vi "Main_24b.vi"() -> ()   [LabVIEW 2020]
uses:
  RB ENUM_Position ID.ctl
  Cluster _Point Location.ctl
  0c90424e-a446-4045-a5ae-fd3bd7481f50.vi
  <vilib>/Comparison/Equal/Equal Functor/Equal Functor.lvclass
panel:
  in  "milliseconds to wait":u32
  in  "Description":string="--- Part Two ---\nAs the expedition reaches the far side of the valley, one of the Elves looks especially dismayed:\n\nHe forgot his snacks at the entrance to the valley!\n\nSince you're so good at dodging blizzards, the Elves humbly request that you go back for his snacks. From the same initial conditions, how quickly can you make it from the start to the goal, then back to the start, then back to the goal?\n\nIn the above example, the first trip to the goal takes 18 minutes, the trip back to the start takes 23 minutes, and the trip back to the goal again takes 13 minutes, for a total time of 54 minutes."
  out "Array":T1[][](array[typedef])
  in  "Example 2":string="#.######\n#>>.<^<#\n#.<..<<#\n#>v.><>#\n#<^v^^>#\n######.#"
  out "Answer":i32
  in  "Puzzle":string="#.######################################################################################################################################################\n#>v<<.^vvv^vv.^^>>v<>><v^<<.>^>v>v<v^vvvvvv^><^<vv<^^^v<vv>vvv.^v>.<>>v^v><<>^<<^vv<<>><<v<v<^v<..^>>vv^><<<v<^^><<<>>>vvv^.^.v>.^v^^.vv>^vv^>^^^><v<<<#\n#.<<v^><<.<>>>>^.<^<^^<>>^.^^.^v<vvv>>vv<^>.>>^^<<<^^>><^><<<v^>v.^^<.<<^v^>^^>.^.v^>.><<vv^>><>^....^<vv^><<^>v<v<^vvv<v<<><^vv<^>v^^^^^^^.^vv<^^<vvv<#\n#<>.v^.v<^><><v^^>>^><.v>^v^vv><><>>^>^v<^>>v^>^vvv^v..>vv>.^vv^<^.<.<v>>^<><v>^>^v..^>^><>vvv<v>^.>>^^<v^v>^<^vv.>.^v><v>v^>.^v<v>.<<vvv><^v^<^<^<vv<>#\n#>v..v^<^^v<><^^>vv>v^^^<^.^<<><^^^v>^<^v<<^>^<<.^><<^>>v^.v.><>>^<<><^^>>v>.^<^<vv><<>..>>v^^^>v>^<vv>.^>^<.^^v<>v>^.^>^^>.^v^>>^v>>>^<<^.^>><>v^>v>v.#\n#>^^^^^v^>>>^^v^v^v>v^v<v^.><<.^..v<^<^<^><<><<<>>v<<>><<^v^^>v>v<>.<vv>^<<<><.v<v<>>v^v<>>^v><.v>><<v><v<vv<<^^<><.^>v>^<^<^>^^.<.v>v^>>>><<<^v.vv<.<>#\n#>vv<vv^v<.<<v><<<^v>v<><vv<<vv<<.^.v>>v>.>v<^<<>v>>vv>..>v<^.v<.^<.>.<<<>>>^v>.^>>>>><<<^>..>>>^<^<>^>><>^><><v>v<<<v^.vvvv<v>>vv^>>>^.v^<>^><.<v>>v>>#\n#>>v.>><v^>v^v.<^.<vvv<<<v<>.^^v<<^^>>^^v^^.^.<>^vv^>>v<>^>v^.vv^v>.v^<>>v<<v<^>^vv^^v^><>v>.^<v<v<.^>>vvv>v^<^vv^<v^<<>^<v<>v<<v<<>v^v><>^vv^<<<^v>^>>#\n#<^<^>><<.<<.><<v>vv>v^v<<>..v<^>v^<.vv><v^<<<.v>v>>><<^.<v^vvv^<^v<<^^^^<v<<.<<^><v.<>>^><v>..<><vvv<.<>><.v>.v><<>vv<>.<<v.>><>>v<v^>^>>..>.<<^>^>^.>#\n#<v.>v>v<>>v^v>^v<^vv>^^>^vv>v<^^vv><^.<v<^<v>^>^v<v.<^<>^>>>vvvv<v>>^^<v.^v<^^<.<<<><v^<>^^<vvv><<>...^<><>^>vvv^^v..v..v^><^<>^>vv><v<^^vv^vvv>v^<v><#\n#<^^^^.>v>><<>v<vv<^<<^>v..vv^vvv>>>v<<^vv^^><^>^>^v.<<^v^^><vv>.>v..v.^v><^<^>>^>vv<<v.v>.<.>^.>>>^>>^^v^>^<.<><v>v^.^..<>.>^<^^<v.^v>^^^<<^v>>.>vv<v>#\n#>^^v>v.<v<<v..>><>..^v><>.^<v.>vv<>v^^>v.^v<<<vv>>v.^>><<^<v><v^.>>>^v>^>>v<<...<^^^vv.v^><<<>^^v<v^>v<v>.vv^vv.>>v<>><>v><vv>^>>v^..vv>v>^^>vvv>.>^v<#\n#<v>^^.<.^vv^<>^vv<<<<<vv^<^^<>v>^vv<>v<<>vv^<<v><<.^^..>.^>vv<^<>>^.<<<<<>.v>v><>.>v>v^<>^>vvv>.<^v^.>^<<v<^vvv^>v><<v^>.^><^><>v.^^<><vv<>.v..^<<v^>>#\n#<>^.>.><><v^<v>v>^<<>^v..<.<><>>^.vv>v.vv.>><>v^>.^><.<v.>v..^^v.^v^>^<^^<>>>v<^>>v<^<v^^^v<^v.vv<v^.><^^v^>^^^<.>.<v<.<v>^.><^^<v^<<^^v<.>>v>.vvv>v>>#\n#<v><v.^^<>v>.>^^^^>v<<v..v>><>v^.>^^<^>v<>v^v<v^<><^<>v>v^.<.^v^<^<>v^^<<^v><^.>^.v><><>>^v^v><.>v><<>v>v^.vvv><>^>>v^<<^v>^vv><><.^^>>vv^^v><^..>^v<>#\n#>v><^<vv^v>v><>v^<<><<^>v^v<^<^<v>><v^vv<<.vv<^v.><<<v.v.^<v<v.^^>><>^vv>v<v^>v^.<<><^<<.<vv<^.^>^^vv<^vv^..<^>^^<^^vvvv<><^^^<v<vv<v^>^v<^v><^^<..<v>#\n#>v^<<><<<^v.vvv>v<<v>>.^>^<^><..>>>^v.v.<<v<>>^^..><<v>vv^^<v<<^<>^v<^<<^.v>^<^>vv.>>>^>^^.<^<v<<^^v^^<><.>^.<><vv^<^>^>>^^vv^<^^^<^>^.v^<.<^^<.>v>v>>#\n#>^<v>v^<^>>..v<.><<<^><^v>vv<>^^v<v^vv><<<><^v<^.v<^>v<v<^<v>v>^v^^>>^<<^.<<v<vvv><^>v>^<>v>v^^>.<vv<<>>^^<>vv>^v^.><^^^vv>v<<<<v^v<vv><.<v<^v>>^v>v<>#\n#<vv^>^^<v>^v>>.^.<<^<^^.v>>vv>^<><><>>^>>>vv<.v<^<<<vvv.>v<>>^>>v<>>..>^v^>^>^v<<>v^v^.^>^v^^v>.><v<<.v<v>vv>>.<<v.v.^<>><>vv>^^>><^^.<>>>vv<<>^>><<<.#\n#<^<^^.>>>^<>^v<^v<<>v^<>^vv<^^v<v<<^^.><<vv>v^<^^<>^^^v<v>^.^^<<^v<v^.^>>>><v>><>>>><v<^^<v>v^v>^>v>v^^^<>v><v><.>><>^vvvvv>vv<<v^^<v^v>v.^v<vv<^.^^v<#\n#..>^>>^^^^v<>>^><^^v>^^>v.><>><vv<><^.<><^v.^vv<><v>v^<<v>v<vv<><>v^.^<<<vv>>^^<<>^.v<^.v^^<>>>^v<.>^..^^^<<<>..v<><v<>v<>>..<v><>^^>>.<>v<<>v>.<v^vv.#\n######################################################################################################################################################.#"
  in  "Example":string="#.#####\n#.....#\n#>....#\n#.....#\n#...v.#\n#.....#\n#####.#"
  # "976"
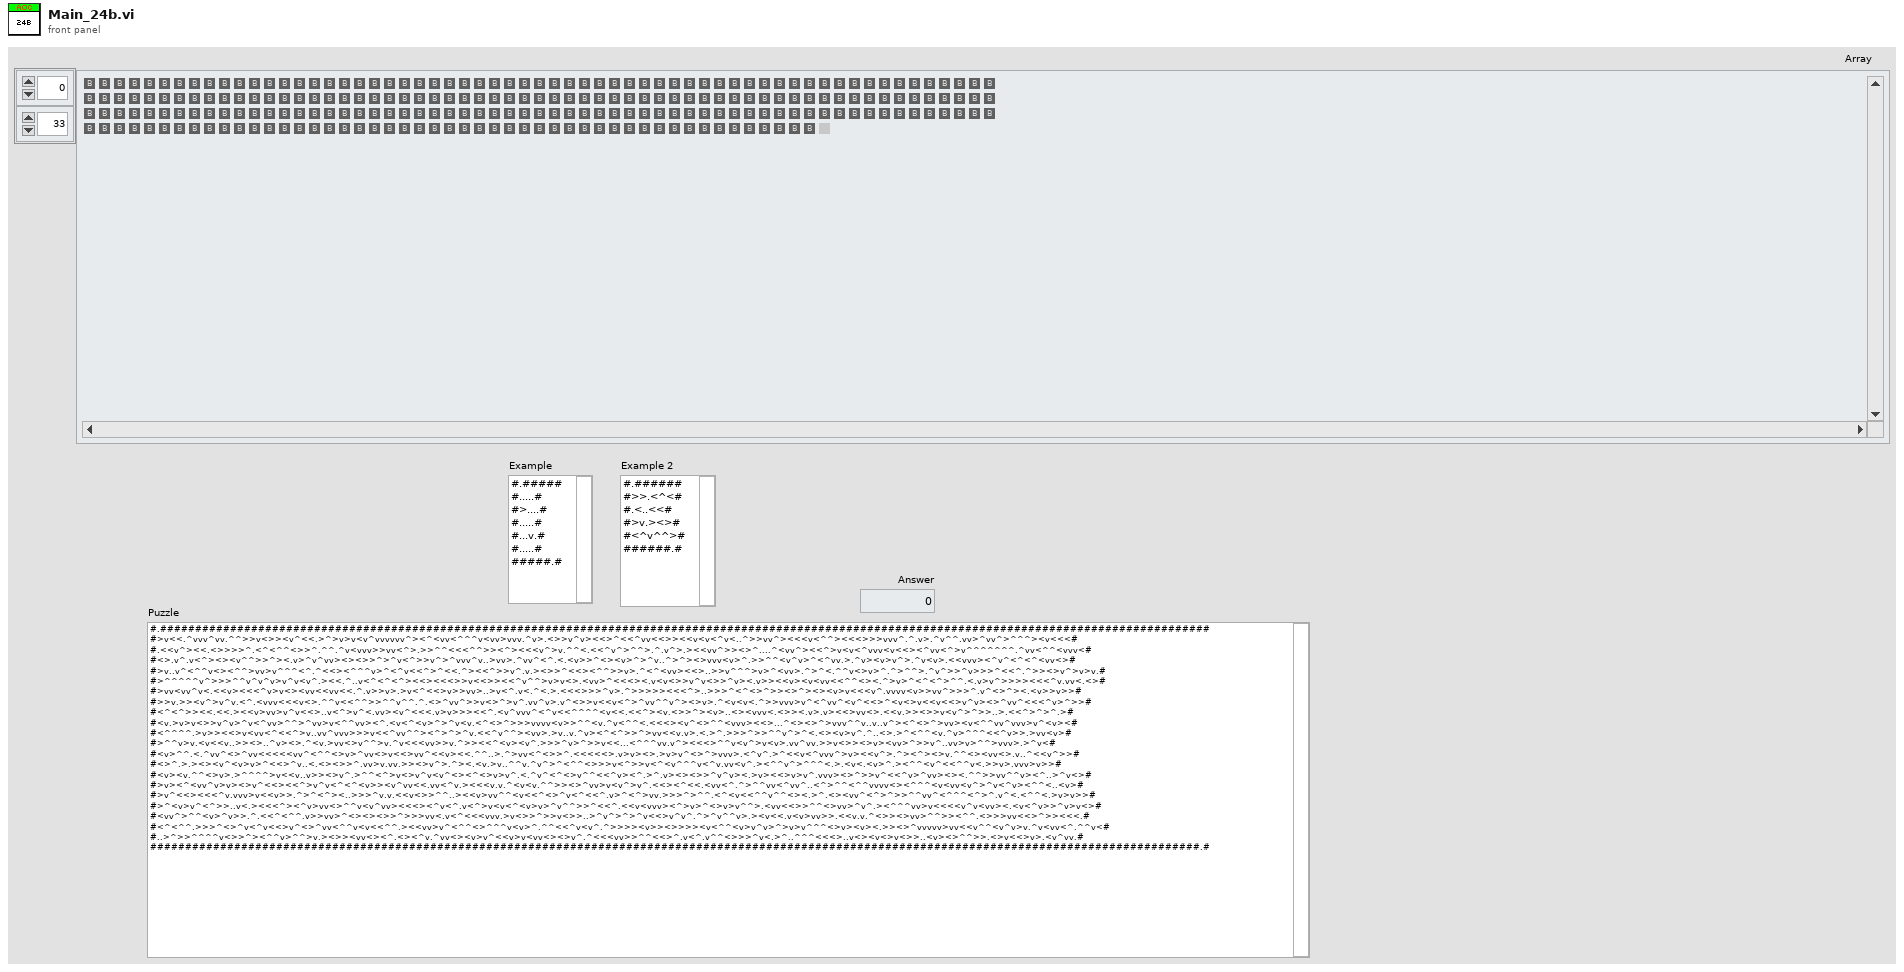
[diagram p1: front panel]
types:
  T1 = typedef "RB ENUM_Position ID.ctl" = enum32{"Blank", "Wall", "UP", "Down", "Left", "Right", "Two", "Three", "Four", "Spot"}
  T2 = typedef "Cluster _Point Location.ctl" = cluster{"X col":i32, "Y row":i32}
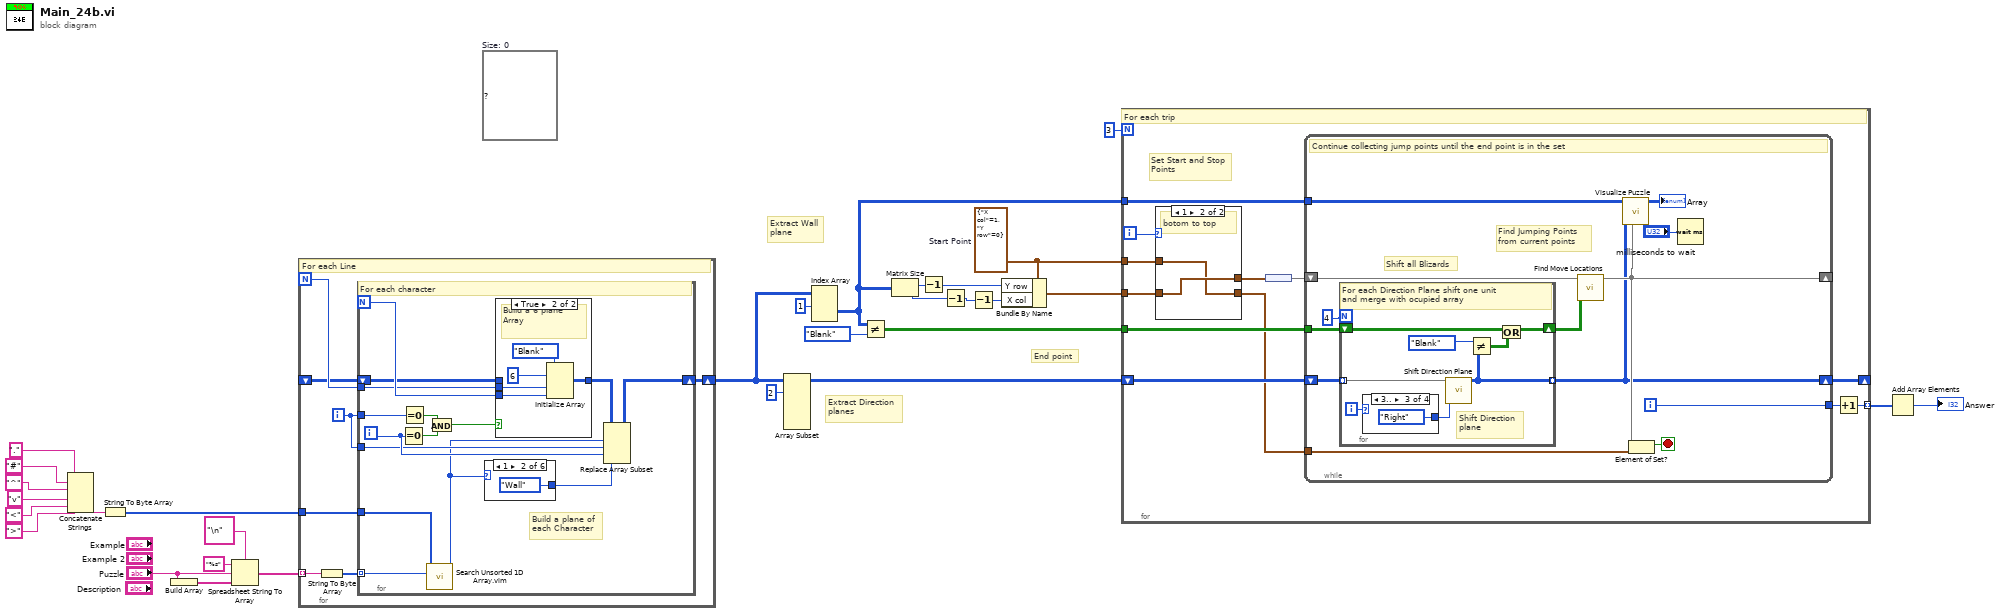
[diagram p0: block diagram]
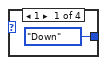
[diagram p3: hidden frame]
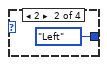
[diagram p4: hidden frame]
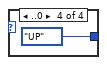
[diagram p5: hidden frame]
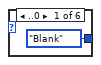
[diagram p6: hidden frame]
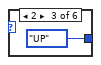
[diagram p7: hidden frame]
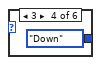
[diagram p8: hidden frame]
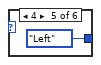
[diagram p9: hidden frame]
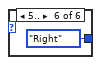
[diagram p10: hidden frame]
diagram:
  w4 = T2 {"X col"=1, "Y row"=0}  # Start Point
  (unwired) map{T2, u32} {}  # Size: 0
  # "End point"
  # "Extract Wall\nplane"
  # "Extract Direction\nplanes"
  n1 = Concatenate Strings(".", "#", "^", "v", "<", ">") -> (w22:string)
  n2 = String To Byte Array(string=w22) -> (unsigned byte array=w21:u8[])
  n3 = Build Array("Puzzle") -> (w30:string[])
  n4 = Spreadsheet String To Array(delimiter (Tab)="\n", format string="%s", spreadsheet string="Puzzle", array type (2D Dbl)=w30) -> (array=w27:string[])
  n5 = for {
    N -> [w35]
    tunnel: w27 -> [w37] mode=indexing
    shift-right: [w34] -> w15
    shift-left: _ -> [w33]
    tunnel: w21 -> [w32]
    i -> [w31]
    # "For each Line"
    n6 = String To Byte Array(string=w37) -> (unsigned byte array=w36:u8[])
    n7 = for {
      N -> [w48]
      tunnel: w36 -> [w43] mode=indexing
      tunnel: w31 -> [w52]
      tunnel: w35 -> [w47]
      shift-right: [w38] -> w34
      shift-left: w33 -> [w46]
      tunnel: w32 -> [w45]
      tunnel: w31 -> [w41]
      i -> [w42]
      # "Build a plane of\neach Character"
      # "For each character"
      n8 = Equal To 0?(x=w42) -> (x = 0?=w50:bool)
      n9 = Equal To 0?(x=w52) -> (x = 0?=w51:bool)
      n10 = call "Search Unsorted 1D Array.vim"("element"=w43, "unsorted 1D array"=w45) -> ("index of element"=w40:i32)  [unwired: 9 in]
      n11 = And(x=w51, y=w50) -> (x .and. y?=w49:bool)
      n12 = case shown="1" w40 {
        tunnel: [RB_ENUM_Position_ID."Blank" ("Position") RB_ENUM_Position_ID."Wall" ("Position") RB_ENUM_Position_ID."UP" ("Position") RB_ENUM_Position_ID."Down" ("Position") RB_ENUM_Position_ID."Left" ("Position") RB_ENUM_Position_ID."Right" ("Position")] -> w39
        frame ..0 {
        }
        frame 1 {
        }
        frame 2 {
        }
        frame 3 {
        }
        frame 4 {
        }
        frame 5.. {
        }
      }
      n13 = case shown="True" w49 {
        tunnel: w48 -> [_ w61]
        tunnel: w47 -> [_ w62]
        tunnel: [w59 w63] -> w44
        tunnel: w46 -> [w59 _]
        frame False {
        }
        frame True {
          # "Build a 6 plane\nArray"
          n14 = Initialize Array(RB_ENUM_Position_ID."Blank" ("Position"), 6 ("dimension size"), w62, w61) -> (w63:T1[][][])
        }
      }
      n15 = Replace Array Subset(array=w44, new element=w39, index (dim 0)=w40, index (dim 1)=w41, index (dim 2)=w42) -> (w38:T1[][][])
    }
  }
  n16 = Array Subset(array=w15, index (dim 0)=2 ("index")) -> (w14:T1[][][])  [unwired: 5 in]
  n17 = Index Array(array=w15, index (dim 0)=1 ("index (page)")) -> (element=w6:T1[][])  [unwired: 2 in]
  n18 = Not Equal?(x=w6, y=RB_ENUM_Position_ID."Blank" ("Position")) -> (x != y?=w12:bool[][])
  n19 = Matrix Size(0:w6) -> (1:w13:i32, 2:w10:i32)
  n20 = Decrement(x=w13) -> (x-1=w8:i32)
  n21 = Decrement(x=w10) -> (x-1=w11:i32)
  n22 = Decrement(x=w11) -> (x-1=w9:i32)
  n23 = Bundle By Name(cluster=w4, "Y row"=w8, "X col"=w9) -> (w7:T2)
  n24 = for {
    N: 3 -> [_]
    tunnel: w12 -> [w75]
    tunnel: w7 -> [w70]
    tunnel: w4 -> [w68]
    tunnel: w6 -> [w73]
    shift-right: [w67] -> _
    shift-left: w14 -> [w76]
    tunnel: [w65] -> w3 mode=indexing
    i -> [w72]
    # "Set Start and Stop\nPoints"
    # "For each trip"
    n25 = case shown="1" w72 {
      tunnel: [w78 w80] -> w71
      tunnel: w70 -> [w77 w80]
      tunnel: [w77 w79] -> w69
      tunnel: w68 -> [w78 w79]
      frame ..0, 2.. {
        # "top to bottom"
      }
      frame 1 {
        # "botom to top"
      }
    }
    n26 = node(w71) -> (w74:set{T2})
    n27 = while {
      shift-right: [w82] -> w67
      shift-left: w76 -> [w93]
      shift-right: [w83] -> _
      shift-left: w74 -> [w88]
      tunnel: w75 -> [w91]
      tunnel: [w89] -> w66
      tunnel: w73 -> [w86]
      tunnel: w69 -> [w84]
      i -> [w89]
      stop <- w90 stop-if-true
      # "Find Jumping Points\nfrom current points"
      # "Shift all Blizards"
      # "Continue collecting jump points until the end point is in the set"
      n28 = for {
        N: 4 -> [_]
        shift-right: [w96] -> w87
        shift-left: w91 -> [w97]
        tunnel: w93 -> [w94] mode=indexing
        tunnel: [w95] -> w82 mode=indexing
        i -> [w101]
        # "Shift Direction\nplane"
        # "For each Direction Plane shift one unit\nand merge with ocupied array"
        n29 = case shown="3.." w101 {
          tunnel: [RB_ENUM_Position_ID."Down" ("Position") RB_ENUM_Position_ID."Left" ("Position") RB_ENUM_Position_ID."Right" ("Position") RB_ENUM_Position_ID."UP" ("Position")] -> w100
          frame 1 {
          }
          frame 2 {
          }
          frame 3.. {
          }
          frame ..0 {
          }
        }
        n30 = call "Shift Direction Plane.vi"("Direction"=w100, "Direction Plane"=w94) -> ("Direction Plane Out"=w95:T1[][])  [unwired: 9 in]
        n31 = Not Equal?(x=RB_ENUM_Position_ID."Blank" ("Position"), y=w95) -> (x != y?=w98:bool[][])
        n32 = Or(x=w97, y=w98) -> (x .or. y?=w96:bool[][])
      }
      n33 = call "Find Move Locations.vi"("Ocupied array"=w87, "Jump Points"=w88) -> ("Jump Points"=w83:set{T2})  [unwired: 9 in]
      n34 = call "Visualize Puzzle.vi"("Jump Points"=w83, "Direction Planes"=w82, "Wall Array"=w86) -> ("Array out"=→"Array":T1[][])  [unwired: 8 in]
      n35 = Element of Set?(10:w84, 11:w83) -> (3:w90:bool)
      n36 = Wait (ms)(milliseconds to wait="milliseconds to wait") -> ()  [unwired: 1 out]
    }
    n37 = Increment(x=w66) -> (x+1=w65:i32)
  }
  n38 = Add Array Elements(numeric array=w3) -> (sum=→"Answer":i32)
